vi "Status_das_Tampas.vi"(0 "Controlador":u16(ring)=3 items=["ZERO", "AH", "DEC", "TUBO", "CUP", "CASS", "COUDE"], 7 "DISPOSITIVO":string="TAMPAS", 11 "Comando":string="LER") -> (3 "Resposta":string="18", 4 "Fechado/Aberto":bool, 6 "Dispositivo Bacia/Centar":bool, 8 "Modo Local/Remoto":bool, 10 "Sistema OFF/ON":bool, 14 "HEXA":u32, 15 "Geral  OFF/ON":bool)   [LabVIEW 2018]
panel:
  out "Erro comunicação":bool
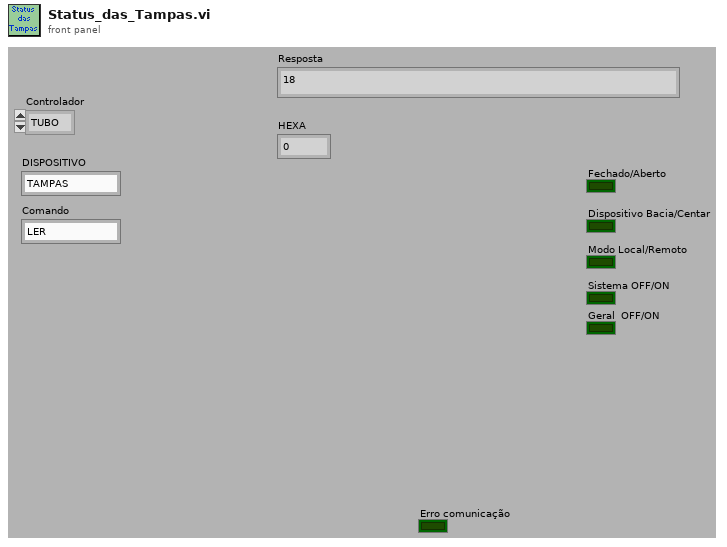
[diagram p1: front panel]
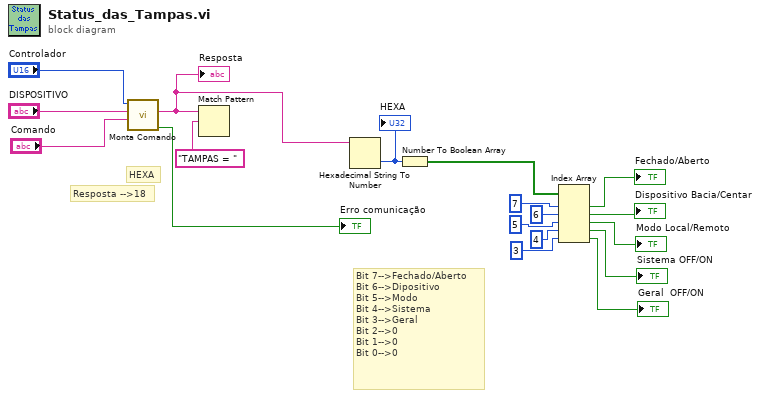
[diagram p0: block diagram]
diagram:
  # "HEXA"
  # "Resposta -->18"
  # "Bit 7-->Fechado/Aberto\nBit 6-->Dipositivo\nBit 5-->Modo\nBit 4-->Sistema\nBit 3-->Geral\nBit 2-->0\nBit 1-->0\nBit 0-->0"
  n1 = call "Monta Comando.vi"("Comando"="Comando", "Dispositivo"="DISPOSITIVO", "Controlador"="Controlador") -> ("Erro Comunicação"=→"Erro comunicação":bool, "Resposta"=w1:string)  [unwired: 4 in, 1 out]
  "Resposta" <- w1
  n2 = Match Pattern(string=w1, regular expression="TAMPAS = ") -> ()  [unwired: 1 in, 4 out]
  n3 = Hexadecimal String To Number(string=w1) -> (number=w7:u32)  [unwired: 2 in, 1 out]
  "HEXA" <- w7
  n4 = Number To Boolean Array(number=w7) -> (Boolean array=w6:bool[])
  n5 = Index Array(array=w6, index #1=7 ("index"), index #2=6 ("index"), index #3=5 ("index"), index #4=4 ("index"), index #5=3 ("index")) -> (element #1=→"Fechado/Aberto":bool, element #2=→"Dispositivo Bacia/Centar":bool, element #3=→"Modo Local/Remoto":bool, element #4=→"Sistema OFF/ON":bool, element #5=→"Geral  OFF/ON":bool)
